vi "circle.vi"(0 "r":dbl) -> (1 "Area":dbl, 2 "Circumference":dbl, 3 "Diameter":dbl)   [LabVIEW 2009]
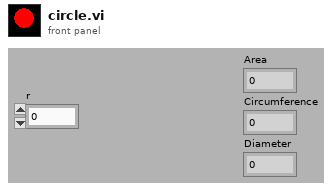
[diagram p1: front panel]
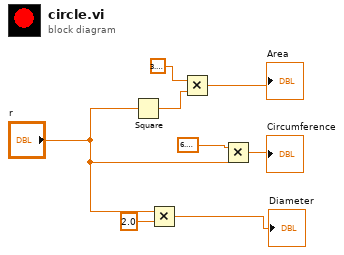
[diagram p0: block diagram]
diagram:
  n1 = Square(x="r") -> (x^2=w4:dbl)
  n2 = Multiply(x="r", y=2.0) -> (x*y=→"Diameter":dbl)
  n3 = Multiply(x=3.141592653589793, y=w4) -> (x*y=→"Area":dbl)
  n4 = Multiply(x=6.283185307179586, y="r") -> (x*y=→"Circumference":dbl)
